vi "hmi_cancel_enable.vi"(7 "hmi_references":T1, 8 "error in (no error)":errorcluster) -> (0 "error out":errorcluster)   [LabVIEW 2015, in "lv-build-interface.lvlib"]
uses:
  lv-build-interface.lvlib
  _controls/hmi_references.ctl
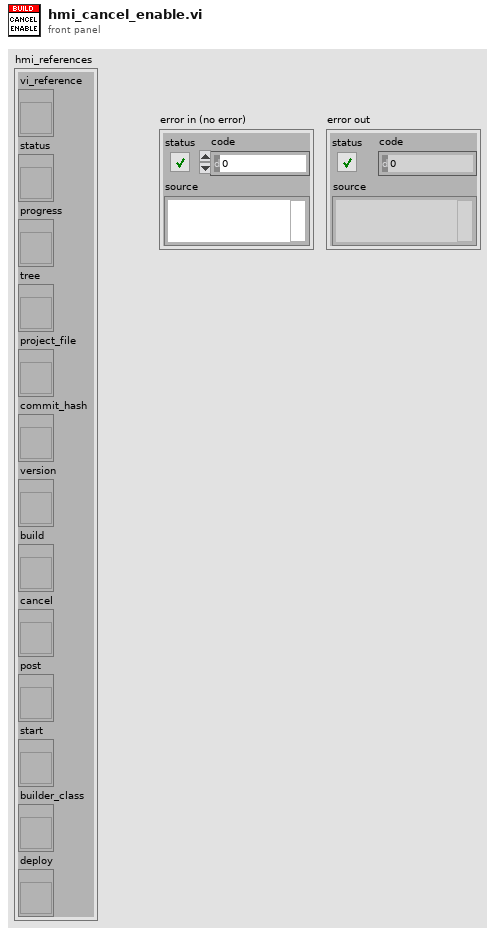
[diagram p1: front panel]
types:
  T1 = typedef "lv-build-interface.lvlib/hmi_references.ctl" = cluster{"vi_reference":refnum<vi>, "status":refnum<vi>, "progress":refnum<vi>, "tree":refnum<vi>, "project_file":refnum<vi>, "commit_hash":refnum<vi>, "version":refnum<vi>, "build":refnum<vi>, "cancel":refnum<vi>, "post":refnum<vi>, "start":refnum<vi>, "builder_class":refnum<vi>, "deploy":refnum<vi>}
  T2 = enum8{"Enabled", "Disabled", "Disabled and Grayed Out"}
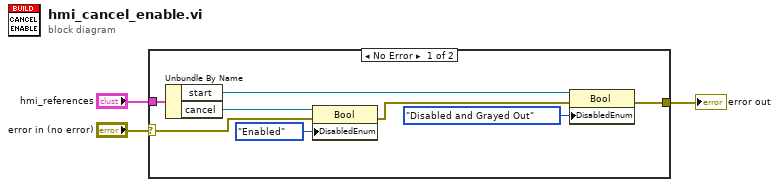
[diagram p0: block diagram]
diagram:
  n1 = case shown="No Error" "error in (no error)" {
    selector: "error in (no error)" -> [w5 w12]
    tunnel: "hmi_references" -> [w7 _]
    tunnel: [w4 w12] -> w1
    frame No Error {
      n2 = Unbundle By Name(w7) -> ("start"=w9:refnum<vi>, "cancel"=w11:refnum<vi>)
      n3 = property class="Bool"(reference=w11, error in=w5, "DisabledEnum"=T2."Enabled" ("Disabled")) -> (error out=w6:errorcluster)  [unwired: 1 out]
      n4 = property class="Bool"(reference=w9, error in=w6, "DisabledEnum"=T2."Disabled and Grayed Out" ("Disabled")) -> (error out=w4:errorcluster)  [unwired: 1 out]
    }
    frame Error {
    }
  }
  "error out" <- w1
